vi "From Variant.vi"(8 "Error In":errorcluster, 10 "Variant":variant, 11 "2D String In":refnum<class "2D String.lvclass">) -> (0 "Error Out":errorcluster, 3 "2D String Out":refnum<class "2D String.lvclass">)   [LabVIEW 2017, in "Tree API.lvlib" / "2D String.lvclass"]
doc: "Dynamic dispatch interface for conversion of variant LV data to Tree Data classes."
uses:
  2D String.lvclass
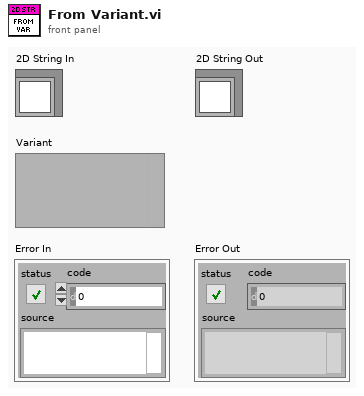
[diagram p1: front panel]
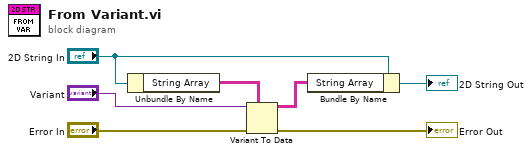
[diagram p0: block diagram]
diagram:
  n1 = Unbundle By Name("2D String In") -> ("String Array"=w4:string[][])
  n2 = Variant To Data(error in="Error In", type=w4, Variant="Variant") -> (data=w3:string[][], error out=→"Error Out":errorcluster)
  n3 = Bundle By Name(cluster="2D String In", "String Array"=w3) -> (→"2D String Out":refnum<class "2D String.lvclass">)
